vi "FlatToRichni_measurementlink_discovery_v1_RegisterServiceRequest.vi"(5 "OutputClusterType":T1, 11 "InputCluster":T5) -> (3 "OutputCluster":T1)   [LabVIEW 2020, in "MeasurementLink Discovery Client.lvlib"]
uses:
  MeasurementLink Discovery Client.lvlib
  ni_measurementlink_discovery_v1_RegisterServiceRequest_Flat.ctl
  ni_measurementlink_discovery_v1_ServiceDescriptor_Flat.ctl
  ni_measurementlink_discovery_v1_ServiceDescriptor_AnnotationsEntry_Flat.ctl
  ni_measurementlink_discovery_v1_ServiceLocation_Flat.ctl
  ni_measurementlink_discovery_v1_RegisterServiceRequest.ctl
  ni_measurementlink_discovery_v1_ServiceDescriptor.ctl
  ni_measurementlink_discovery_v1_ServiceDescriptor_AnnotationsEntry.ctl
  ni_measurementlink_discovery_v1_ServiceLocation.ctl
  FlatToRichni_measurementlink_discovery_v1_ServiceDescriptor_AnnotationsEntry.vi
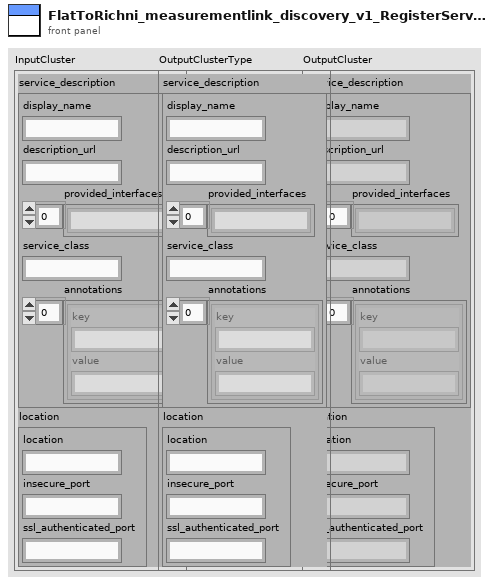
[diagram p1: front panel]
types:
  T1 = typedef "MeasurementLink Discovery Client.lvlib/ni_measurementlink_discovery_v1_RegisterServiceRequest.ctl" = cluster{"service_description":T2, "location":T4}
  T2 = typedef "MeasurementLink Discovery Client.lvlib/ni_measurementlink_discovery_v1_ServiceDescriptor.ctl" = cluster{"display_name":string, "description_url":string, "provided_interfaces":string[], "service_class":string, "annotations":T3[]}
  T3 = typedef "MeasurementLink Discovery Client.lvlib/ni_measurementlink_discovery_v1_ServiceDescriptor_AnnotationsEntry.ctl" = cluster{"key":string, "value":string}
  T4 = typedef "MeasurementLink Discovery Client.lvlib/ni_measurementlink_discovery_v1_ServiceLocation.ctl" = cluster{"location":string, "insecure_port":string, "ssl_authenticated_port":string}
  T5 = typedef "MeasurementLink Discovery Client.lvlib/ni_measurementlink_discovery_v1_RegisterServiceRequest_Flat.ctl" = cluster{"service_description":T6, "location":T8}
  T6 = typedef "MeasurementLink Discovery Client.lvlib/ni_measurementlink_discovery_v1_ServiceDescriptor_Flat.ctl" = cluster{"display_name":string, "description_url":string, "provided_interfaces":string[], "service_class":string, "annotations":T7[]}
  T7 = typedef "MeasurementLink Discovery Client.lvlib/ni_measurementlink_discovery_v1_ServiceDescriptor_AnnotationsEntry_Flat.ctl" = cluster{"key":string, "value":string}
  T8 = typedef "MeasurementLink Discovery Client.lvlib/ni_measurementlink_discovery_v1_ServiceLocation_Flat.ctl" = cluster{"location":string, "insecure_port":string, "ssl_authenticated_port":string}
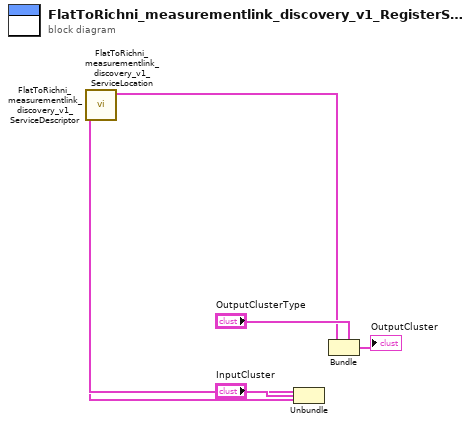
[diagram p0: block diagram]
diagram:
  n1 = Unbundle "Unbundle"("InputCluster") -> ("service_description"=w4:T6, "location"=w2:T8)
  n2 = call "FlatToRichni_measurementlink_discovery_v1_ServiceLocation.vi"("InputCluster"=w2) -> ("OutputCluster"=w1:T4)  [unwired: 10 in]
  n3 = call "FlatToRichni_measurementlink_discovery_v1_ServiceDescriptor.vi"("InputCluster"=w4) -> ("OutputCluster"=w3:T2)  [unwired: 10 in]
  n4 = Bundle "Bundle"(cluster="OutputClusterType", "service_description"=w3, "location"=w1) -> (→"OutputCluster":T1)
